vi "1kclass_1dt.vi"() -> (0 "max jitter (uS)":dbl format="%.2f", 1 "mean time (uS)":dbl format="%.2f", 2 "standard deviation (uS)":dbl format="%.2f", 3 "execution histogram":T1(graph), 4 "Error":errorcluster, 5 "execution times (uS)":dbl[](graph))   [LabVIEW 2013]
uses:
  standard timing source/ms timing source.lvclass
  <vilib>/Platform/TimedLoop/XDataNode/timing_clust.ctl
  <vilib>/Platform/TimedLoop/XDataNode/nitl_modes.ctl
  <vilib>/Platform/TimedLoop/XDataNode/wakeup.ctl
  <vilib>/platform/TimedLoop/XDataNode/XDataNode.xnode
  <vilib>/Platform/TimedLoop/XDataNode/XDNodeRunTimeDep.lvlib
panel:
  out "x-y":i64
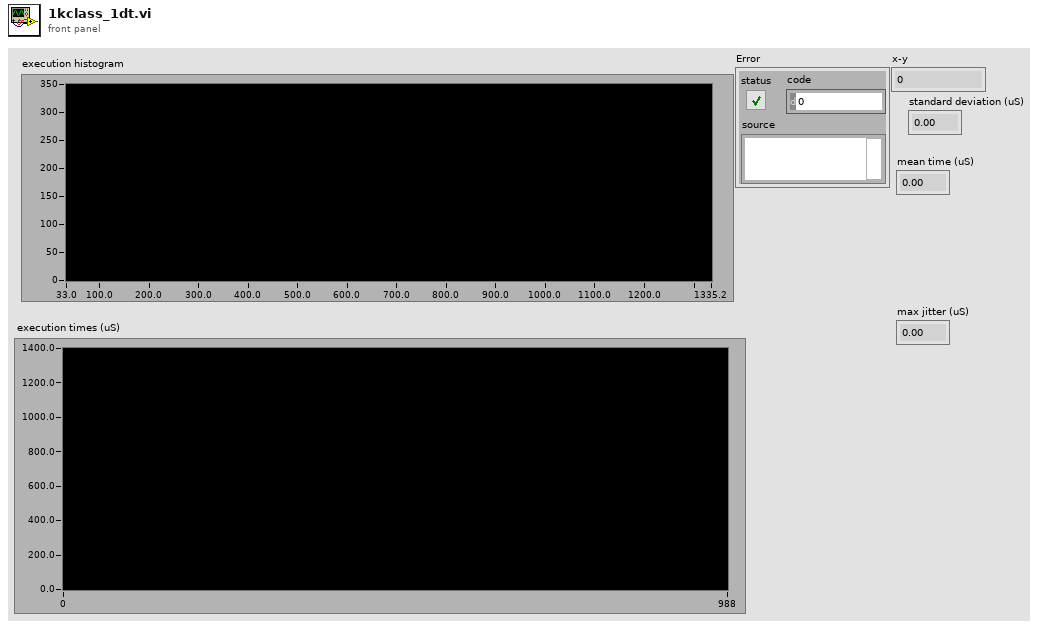
[diagram p1: front panel]
types:
  T1 = cluster{"X Values":dbl[], "Histogram: h(x)":i32[]}
  T2 = typedef "XDNodeRunTimeDep.lvlib/timing_clust.ctl" = cluster{"Expected End [f-1]":u64, "Actual End [f-1]":u64, "Finished Late? [f-1]":bool, "Expected End [i-1]":u64, "Actual End [i-1]":u64, "Finished Late? [i-1]":bool, "Expected Start [i]":u64, "Actual Start [i]":u64, "Expected Start [f]":u64, "Actual Start [f]":u64, "Source Name":string, "Structure Name":string, "Period":i64, "Deadline":i64, "Offset":i64, "Start":i64, "Priority":i32, "Timeout":i32, "Mode":T3, "Wakeup Reason":T4, "Error":errorcluster, "Source Type":string, "Secondary Source Type":string, "Global End Time":u64, "Global Start Time":u64, "Frame Duration":u64, "Iteration Duration":u64, "Assigned CPU":i32, "I/O Scan Engine Mode":u32}
  T3 = typedef "XDNodeRunTimeDep.lvlib/nitl_modes.ctl" = enum32{"No Change", "Process missed periods, maintain original phase", "Discard missed periods, maintain original phase", "Process missed periods, ignore original phase", "Discard missed periods, ignore original phase"}
  T4 = typedef "XDNodeRunTimeDep.lvlib/wakeup.ctl" = enum32{"Normal", "Aborted", "Asynchronous wakeup", "Timing source error", "Timed loop error", "Timeout"}
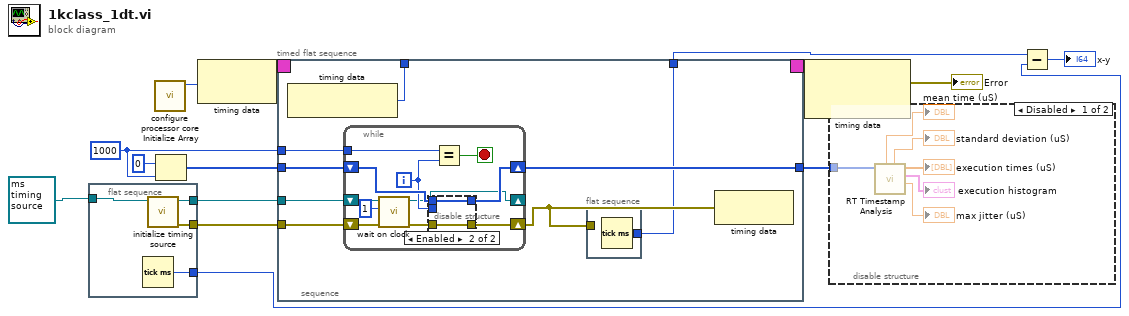
[diagram p0: block diagram]
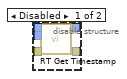
[diagram p3: hidden frame]
diagram:
  w12 = 1000 ("x")
  n1 = flat-sequence {
    tunnel: refnum<class "ms timing source.lvclass"> refnum ("ms timing source.lvclass") -> [w18]
    tunnel: [w17] -> w5
    tunnel: [w16] -> w4
    tunnel: [w15] -> w1
    frame #0 {
      n2 = Tick Count (ms)() -> (millisecond timer value=w15:u32)
      n3 = call-dynamic "initialize timing source.vi"("timing source in"=w18) -> ("error out"=w16:errorcluster, "timing source out"=w17:refnum<class "ms timing source.lvclass">)  [unwired: 9 in]
    }
  }
  n4 = call "configure processor core.vi"() -> ("Processor"=w7:i32)  [unwired: 11 in]
  n5 = Initialize Array(u64 0, w12) -> (w13:u64[])
  n6 = node-c288(w7) -> (w10:T2)
  n7 = timed-sequence {
    timing: w10 -> [_]
    timing-out: [_] -> w9
    tunnel: w12 -> [w25]
    tunnel: w13 -> [w24]
    tunnel: [w23] -> w11
    tunnel: w5 -> [w22]
    tunnel: w4 -> [w21]
    tunnel: [w20] -> _
    tunnel: [w19] -> w2
    n8 = timed-flat-sequence {
      tunnel: w25 -> [w33]
      tunnel: w24 -> [w32]
      tunnel: [w31] -> w23
      tunnel: w22 -> [w30]
      tunnel: w21 -> [w29]
      tunnel: [w28] -> w20
      tunnel: [w26] -> w19
      n9 = node-c288() -> (w28:i64)  [unwired: 1 in]
      n10 = while {
        tunnel: w33 -> [w45]
        shift-right: [w43] -> w31
        shift-left: w32 -> [w44]
        shift-right: [w38] -> _
        shift-left: w30 -> [w39]
        shift-right: [w37] -> w27
        shift-left: w29 -> [w36]
        i -> [w41]
        stop <- w42 stop-if-true
        n11 = call-dynamic "wait on clock.vi"("error in"=w36, "dt"=u32 1, "timing source in"=w39) -> ("error out"=w40:errorcluster, "timing source out"=w38:refnum<class "ms timing source.lvclass">)  [unwired: 6 in, 1 out]
        n12 = disable-structure shown="Enabled" {
          disable-tunnel: w44 -> [w50 w52]
          disable-tunnel: [w49 w52] -> w43
          disable-tunnel: w41 -> [w48 _]
          disable-tunnel: w40 -> [w47 w51]
          disable-tunnel: [w46 w51] -> w37
          frame Disabled {
            n13 = call <vilib>:"RT Get Timestamp.vi"("error in (no error)"=w47, "iteration"=w48, "timestamp array in"=w50) -> ("error out"=w46:errorcluster, "timestamp array out"=w49:u64[])  [unwired: 7 in]
          }
          frame Enabled {
          }
        }
        n14 = Equal?(x=w45, y=w41) -> (x = y?=w42:bool)
      }
      n15 = flat-sequence {
        tunnel: w27 -> [_]
        tunnel: [w34] -> w26
        frame #0 {
          n16 = Tick Count (ms)() -> (millisecond timer value=w34:u32)
        }
      }
      n17 = node-c288(w27) -> ()  [unwired: 1 out]
    }
  }
  n18 = node-c288(w9) -> (→"Error":errorcluster)  [unwired: 1 out]
  n19 = disable-structure shown="Disabled" {
    disable-tunnel: w11 -> [w63 _]
    frame Disabled {
      n20 = call <vilib>:"RT Timestamp Analysis.vi"("timestamp array"=w63) -> ("max jitter (uS)"=→"max jitter (uS)":dbl, "execution histogram"=→"execution histogram":T1, "execution times (uS)"=→"execution times (uS)":dbl[], "standard deviation (uS)"=→"standard deviation (uS)":dbl, "mean time (uS)"=→"mean time (uS)":dbl)  [unwired: 5 in, 1 out]
    }
    frame Enabled {
    }
  }
  n21 = Subtract(x=w2, y=w1) -> (x-y=→"x-y":u32)
